vi "Leap Screen Tap Gesture.vi"() -> ()   [LabVIEW 2011, in "LMH-Leap.lvlib"]
doc: "This example demonstrates how to read the position of a screen tap gesture using the Leap Motion Controller."
uses:
  vi.lib/MakerHub/Leap/LMH-Leap.lvlib
  vi.lib/MakerHub/Leap/Public/Gestures/Screen Tap/Instance VIs/Read 1 Screen Tap Position.vi
panel:
  out "Last Screen Tap Position":cluster{"X":sgl, "Y":sgl, "Z":sgl}
  out "X Y Screen Tap Position":cluster{"X":sgl, "Z":sgl}[](graph)
  in  "Stop Button":bool
  # "Leap Screen Tap Gesture Example\n\nThis example demonstrates how to read the position of a screen tap gesture using the Leap Motion Controller.\n\nInstructions\n1. Connect the Leap Motion Controller to the host computer.\n2. Click the Run Arrow.\n3. Make a screen tap gesture above the Leap and notice the position indicated on the graph below."
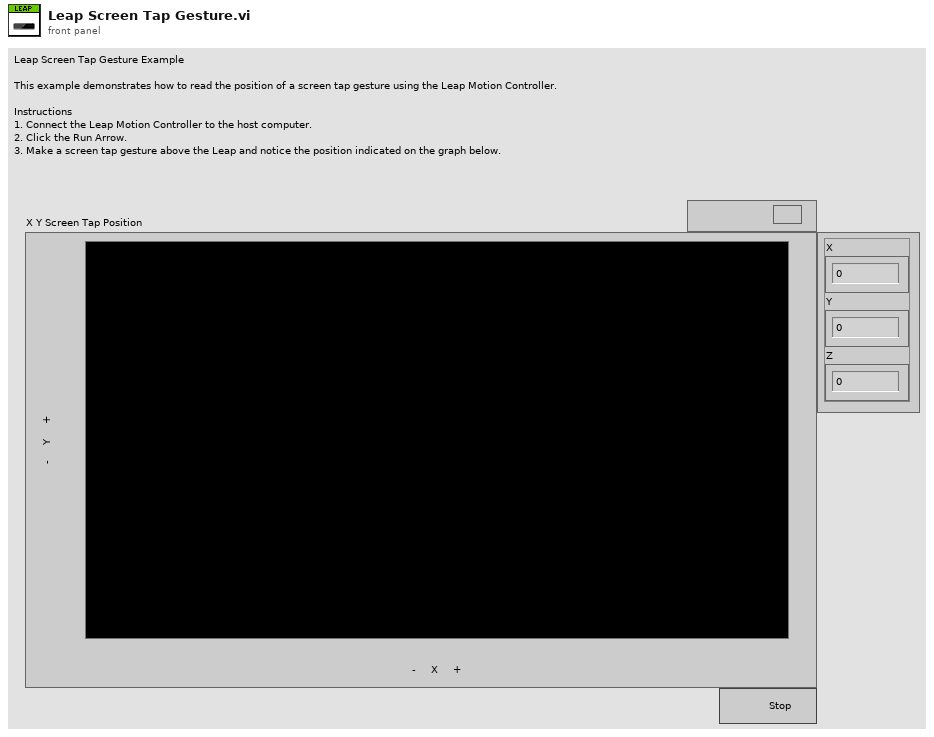
[diagram p1: front panel]
types:
  T1 = typedef "LMH-Leap.lvlib/Leap Handle.ctl" = cluster{"LeapCSharp":refnum<k24>}
  T2 = typedef "LMH-Leap.lvlib/Gesture State.ctl" = enum16{"Invalid", "Start", "Update", "Stop"}
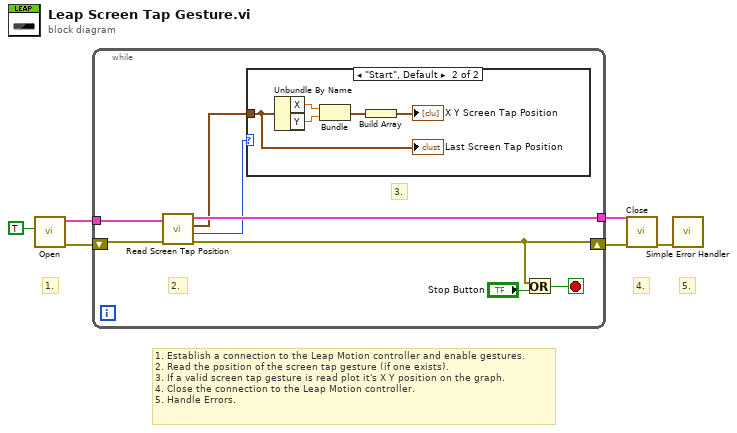
[diagram p0: block diagram]
diagram:
  # "5."
  # "4."
  # "1."
  # "1. Establish a connection to the Leap Motion controller and enable gestures.\n2. Read the position of the screen tap gesture (if one exists).\n3. If a valid screen tap gesture is read plot it's X Y position on the graph.\n4. Close the connection to the Leap Motion controller.\n5. Handle Errors."
  n1 = call "Open.vi"("Enable Gestures? (T)"=TRUE) -> ("Error Out"=w4:errorcluster, "Leap Handle"=w6:T1)  [unwired: 9 in]
  n2 = while {
    tunnel: w6 -> [w12]
    shift-right: [w7] -> w5
    shift-left: w4 -> [w11]
    tunnel: [w10] -> w1
    stop <- w14 stop-if-true
    # "3."
    # "2."
    n3 = call-poly "Read Screen Tap Position.vi"("Error In"=w11, "Leap Handle"=w12) -> ("Error Out"=w7:errorcluster, "Screen Tap Status"=w8:T2, "Screen Tap Position"=w9:cluster{"X":sgl, "Y":sgl, "Z":sgl}, "Leap Handle"=w10:T1)  [unwired: 6 in]
    n4 = case shown="\"Start\", Default" w8 {
      tunnel: w9 -> [_ w19]
      frame "Invalid" {
      }
      frame "Start", Default {
        n5 = Unbundle By Name(w19) -> ("X"=w18:sgl, "Y"=w17:sgl)
        n6 = Bundle("X"=w18, "Y"=w17) -> (w16:cluster{"X":sgl, "Y":sgl})  [unwired: 1 in]
        n7 = Build Array(w16) -> (→"X Y Screen Tap Position":cluster{"X":sgl, "Y":sgl}[])
        "Last Screen Tap Position" <- w19
      }
    }
    n8 = Or(x=w7, y="Stop Button") -> (x .or. y?=w14:bool)
  }
  n9 = call "Close.vi"("Error In"=w5, "Leap Handle"=w1) -> ("Error Out"=w2:errorcluster)  [unwired: 9 in]
  n10 = call <vilib>:"Simple Error Handler.vi"("error in (no error)"=w2) -> ()  [unwired: 4 in, 5 out]
